vi "Square.vi"() -> ()   [LabVIEW 2016, in "SimpleCalculator.lvlib"]
uses:
  SimpleCalculator.lvlib
panel:
  in  "Cancel":bool
  in  "OK":bool
  out "Output":dbl
  in  "Input":dbl
  # "Square"
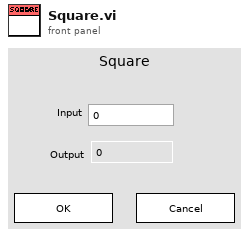
[diagram p1: front panel]
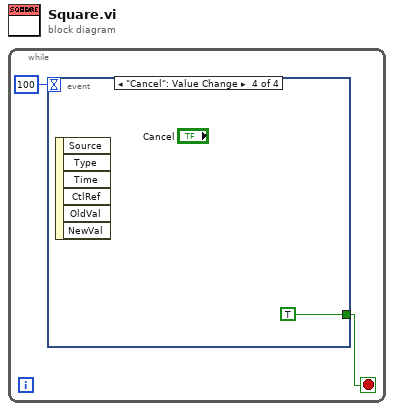
[diagram p0: block diagram]
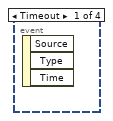
[diagram p2: hidden frame]
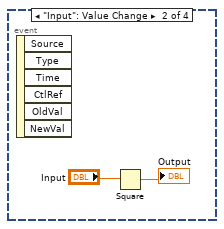
[diagram p3: hidden frame]
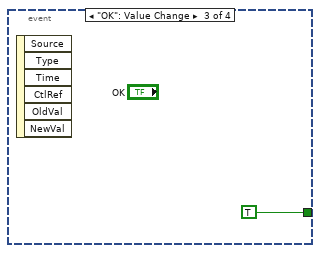
[diagram p4: hidden frame]
diagram:
  n1 = while {
    stop <- w1 stop-if-true
    n2 = event shown="[3] \"Cancel\": Value Change" {
      selector: _ -> [_ _ _ _]
      dyn-events: _ -> [_ _ _ _]
      timeout: 100 -> [_ _ _ _]
      tunnel: [_ _ TRUE TRUE] -> w1
      event Timeout {
        n3 = event-data() -> ()  [unwired: 1 in, 3 out]
      }
      event "Input": Value Change {
        n4 = event-data() -> ()  [unwired: 1 in, 6 out]
        n5 = Square(x="Input") -> (x^2=→"Output":dbl)
      }
      event "OK": Value Change {
        n6 = event-data() -> ()  [unwired: 1 in, 6 out]
      }
      event "Cancel": Value Change {
        n7 = event-data() -> ()  [unwired: 1 in, 6 out]
      }
    }
  }
